vi "DoSomething.vi"(6 "timeout in ms (-1)":i32=-1, 8 "error in (no error)":errorcluster, 10 "Msg":string, 11 "NewTemplate in":refnum<class "Shell.lvclass">) -> (0 "error out":errorcluster, 1 "timed out?":bool, 2 "Value":dbl, 3 "NewTemplate out":refnum<class "Shell.lvclass">)   [LabVIEW 2024, in "Shell.lvclass"]
uses:
  Shell.lvclass
  Shell.lvclass/Shell.ctl
  RQMHCore/ModuleCore/RQMHModule.lvclass
  RQMHCore/ModuleCore/Reply.ctl
  Do Something Args.ctl
  Do Something ReplyArgs.ctl
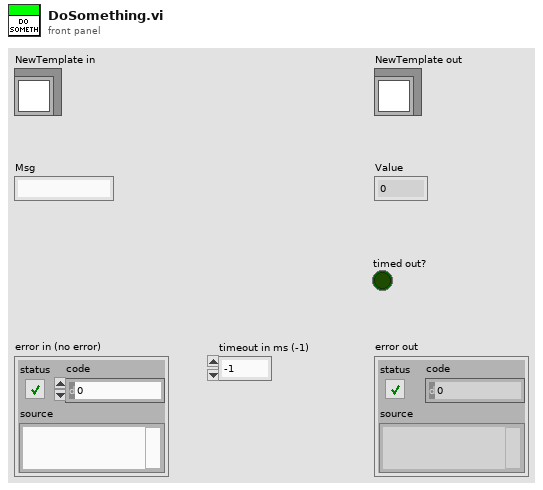
[diagram p1: front panel]
types:
  T1 = typedef "RQMHModule.lvclass/Reply.ctl" = cluster{"Expects Reply":bool, "Reply":refnum<notifier>}
  T2 = typedef "Shell.lvclass/Do Something Args.ctl" = cluster{"Msg":string}
  T3 = typedef "Shell.lvclass/Do Something ReplyArgs.ctl" = cluster{"Value":dbl, "Boolean":bool}
  T4 = cluster{"RQMH_REPLYARGS":T3, "error in (no error)":errorcluster}
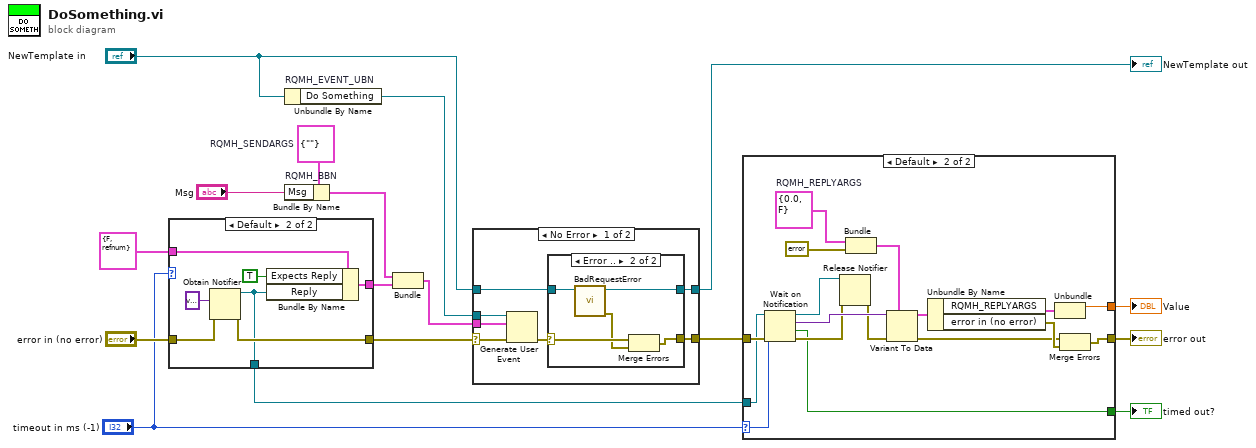
[diagram p0: block diagram]
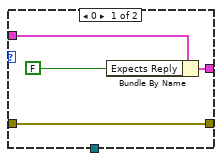
[diagram p4: hidden frame]
diagram:
  w11 = T2 {"Msg"=""}  # RQMH_SENDARGS
  n1 = case shown="Default" "timeout in ms (-1)" {
    tunnel: [w20 w27] -> w13
    tunnel: "error in (no error)" -> [w18 w26]
    tunnel: [w18 w25] -> w8
    tunnel: [_ w24] -> w6
    tunnel: T1 {"Expects Reply"=FALSE, "Reply"=refnum} ("Reply") -> [w21 w23]
    frame 0 {
      n2 = Bundle By Name(cluster=w21, "Expects Reply"=FALSE) -> (w20:T1)
    }
    frame Default {
      n3 = Obtain Notifier(notification data type=variant, error in (no error)=w26) -> (notifier out=w24:refnum<notifier>, error out=w25:errorcluster)  [unwired: 2 in, 1 out]
      n4 = Bundle By Name(cluster=w23, "Expects Reply"=TRUE, "Reply"=w24) -> (w27:T1)
    }
  }
  n5 = Unbundle By Name "RQMH_EVENT_UBN"("NewTemplate in") -> ("Do Something"=w17:refnum<user-event>)
  n6 = Bundle By Name "RQMH_BBN"(cluster=w11, "Msg"="Msg") -> (w14:T2)
  n7 = Bundle("RQMH_SENDARGS"=w14, "Reply"=w13) -> (w12:cluster{"RQMH_SENDARGS":T2, "Reply":T1})  [unwired: 1 in]
  n8 = case shown="No Error" w8 {
    selector: w8 -> [w32 w43]
    tunnel: w12 -> [w35 _]
    tunnel: w17 -> [w34 _]
    tunnel: [w31 w43] -> w7
    tunnel: "NewTemplate in" -> [w30 w44]
    tunnel: [w29 w44] -> w15
    frame No Error {
      n9 = Generate User Event(user event=w34, event data cluster=w35, error in=w32) -> (error out=w33:errorcluster)  [unwired: 1 in, 1 out]
      n10 = case shown="Error .." w33 {
        selector: w33 -> [w36 w42]
        tunnel: [w36 w41] -> w31
        tunnel: w30 -> [w37 w40]
        tunnel: [w37 w39] -> w29
        frame No Error {
        }
        frame Error {
          n11 = call "BadRequestError.vi"("JQMHModule in"=w40) -> ("error out"=w38:errorcluster, "JQMHModule out"=w39:refnum<class "Shell.lvclass">)  [unwired: 9 in]
          n12 = Merge Errors(w42, w38) -> (w41:errorcluster)
        }
      }
    }
    frame Error {
    }
  }
  "NewTemplate out" <- w15
  n13 = case shown="Default" "timeout in ms (-1)" {
    selector: "timeout in ms (-1)" -> [_ w46]
    tunnel: w7 -> [w45 w62]
    tunnel: w6 -> [_ w61]
    tunnel: [w45 w53] -> w5
    tunnel: [_ w49] -> w4
    tunnel: [_ w47] -> w3
    frame 0 {
    }
    frame Default {
      w60 = T3 {"Value"=0.0, "Boolean"=FALSE}  # RQMH_REPLYARGS
      n14 = Wait on Notification(notifier=w61, timeout in ms (-1)=w46, error in (no error)=w62) -> (notifier out=w52:refnum<notifier>, notification=w57:variant, timed out?=w49:bool, error out=w51:errorcluster)  [unwired: 1 in]
      n15 = Release Notifier(notifier=w52, error in (no error)=w51) -> (error out=w50:errorcluster)  [unwired: 1 in, 2 out]
      n16 = Bundle("RQMH_REPLYARGS"=w60, "error in (no error)"=errorcluster {"status"=FALSE, "code"=0, "source"=""}) -> (w59:T4)  [unwired: 1 in]
      n17 = Variant To Data(error in=w50, type=w59, Variant=w57) -> (data=w56:T4, error out=w54:errorcluster)
      n18 = Unbundle By Name(w56) -> ("RQMH_REPLYARGS"=w48:T3, "error in (no error)"=w55:errorcluster)
      n19 = Unbundle(w48) -> ("Value"=w47:dbl)  [unwired: 1 out]
      n20 = Merge Errors(w54, w55) -> (w53:errorcluster)
    }
  }
  "error out" <- w5
  "timed out?" <- w4
  "Value" <- w3
